vi "Define Schema Name.vi"(11 "Sequence Context":T1) -> (0 "error out":errorcluster, 3 "SchemaName":string)   [LabVIEW 2023, in "HardwareAbstractionLayer_LVOOP.lvlib" / "Report.lvclass"]
uses:
  Report.lvclass
  <vilib>/addons/TestStand/_TSLegacy.llb/LabVIEW Test - Sequence Context.ctl
  Control/Action FGV.ctl
  Control/Result FGV Data.ctl
  <vilib>/Utility/error.llb/Trim Whitespace One-Sided.vi
  <vilib>/addons/TestStand/_TSUtility.llb/TestStand - Get Property Value (String).vi
  <vilib>/addons/TestStand/_TSUtility.llb/TestStand - Set Property Value (String).vi
  <vilib>/addons/TestStand/_TSUtility.llb/TestStand - Set Property Value (Number {Unsigned 32-bit Integer}).vi
  Database/Database.lvclass
  Database/SQL Public VI/Control/DB Options.ctl
panel:
  out "# Total Cycles":u32
  out "# Cycles Completed":u32
  in  "Schema":string(combo)
  in  "Temparature Chamber Name":string
  in  "Test Description":string
  in  "Project Name":string
  out "Date and Time":string
  out "current time":timestamp
  in  "Ok":bool
  in  "Test Phase":string(combo)
  in  "Test Name":string(combo)
  in  "Product Varient":string(combo)
  in  "Product Name":string(combo)
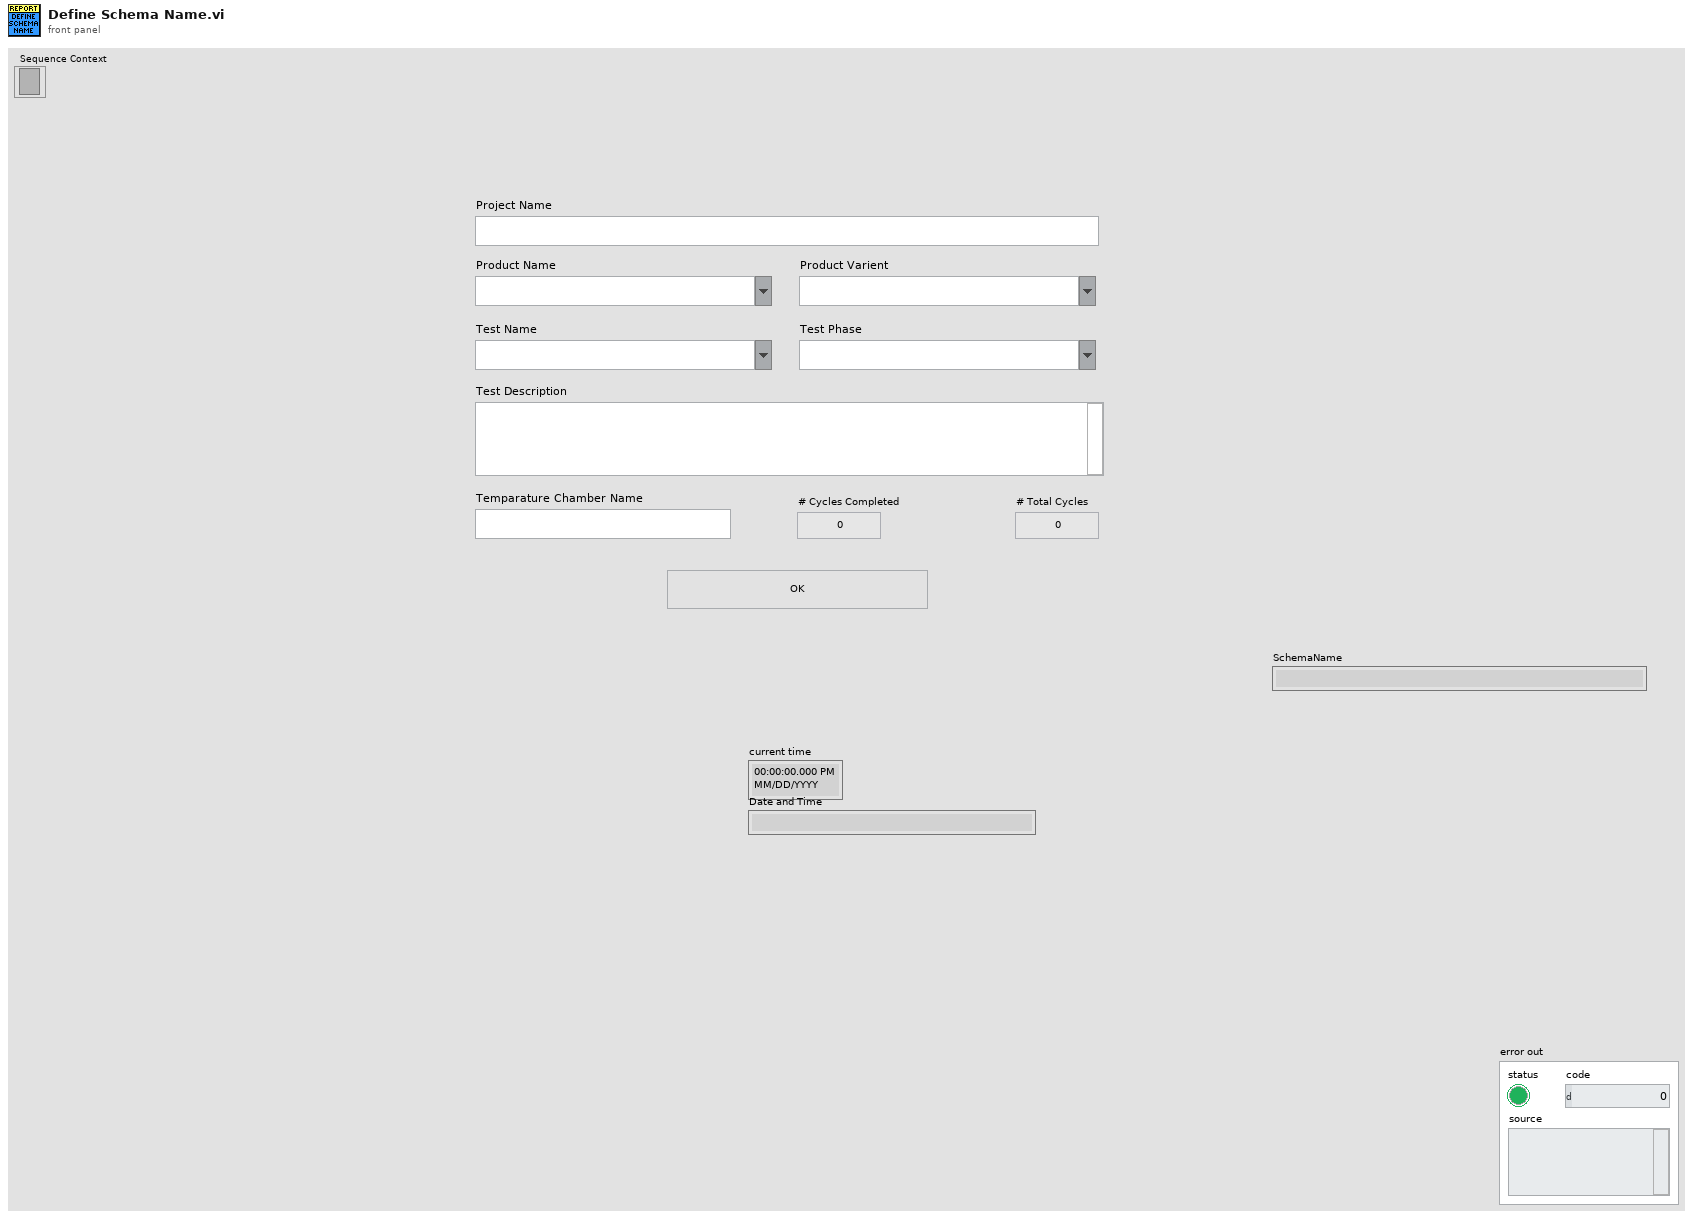
[diagram p1: front panel]
types:
  T1 = typedef "LabVIEW Test - Sequence Context.ctl" = refnum<k7>
  T2 = typedef "HardwareAbstractionLayer_LVOOP.lvlib/Database.lvclass/DB Options.ctl" = enum16{"Init", "Select Data", "Insert Data", "Update Data", "Delete Data", "Execute Query", "Create Schema", "Create Table", "List Tables", "List Columns", "Close"}
  T3 = enum8{"Enabled", "Disabled", "Disabled and Grayed Out"}
  T4 = typedef "HardwareAbstractionLayer_LVOOP.lvlib/Report.lvclass/Result FGV Data.ctl" = cluster{"Project Name":string, "Product Name":string, "Product Varient":string, "Test Name":string, "Test Phase":string, "Test Description":string, "Temp Chamber Name":string, "Schema":string, "Total No of Cycles":u32, "Current Cycle Number":u32, "Cycle Duration":u32, "Current Test Mode":string}
  T5 = typedef "HardwareAbstractionLayer_LVOOP.lvlib/Report.lvclass/Action FGV.ctl" = enum16{"Init", "Set Project Name", "Set Product Name", "Set Product Varient", "Set Test Name", "Set Test Phase", "Set Test Description", "Set Temp Chamber Name", "Set Cycle Duration", "Set Current Cycle Number", "Set Schema", "Set Total No Of Cycle", "Set Current Test Mode", "Set All Data", "Get All Data"}
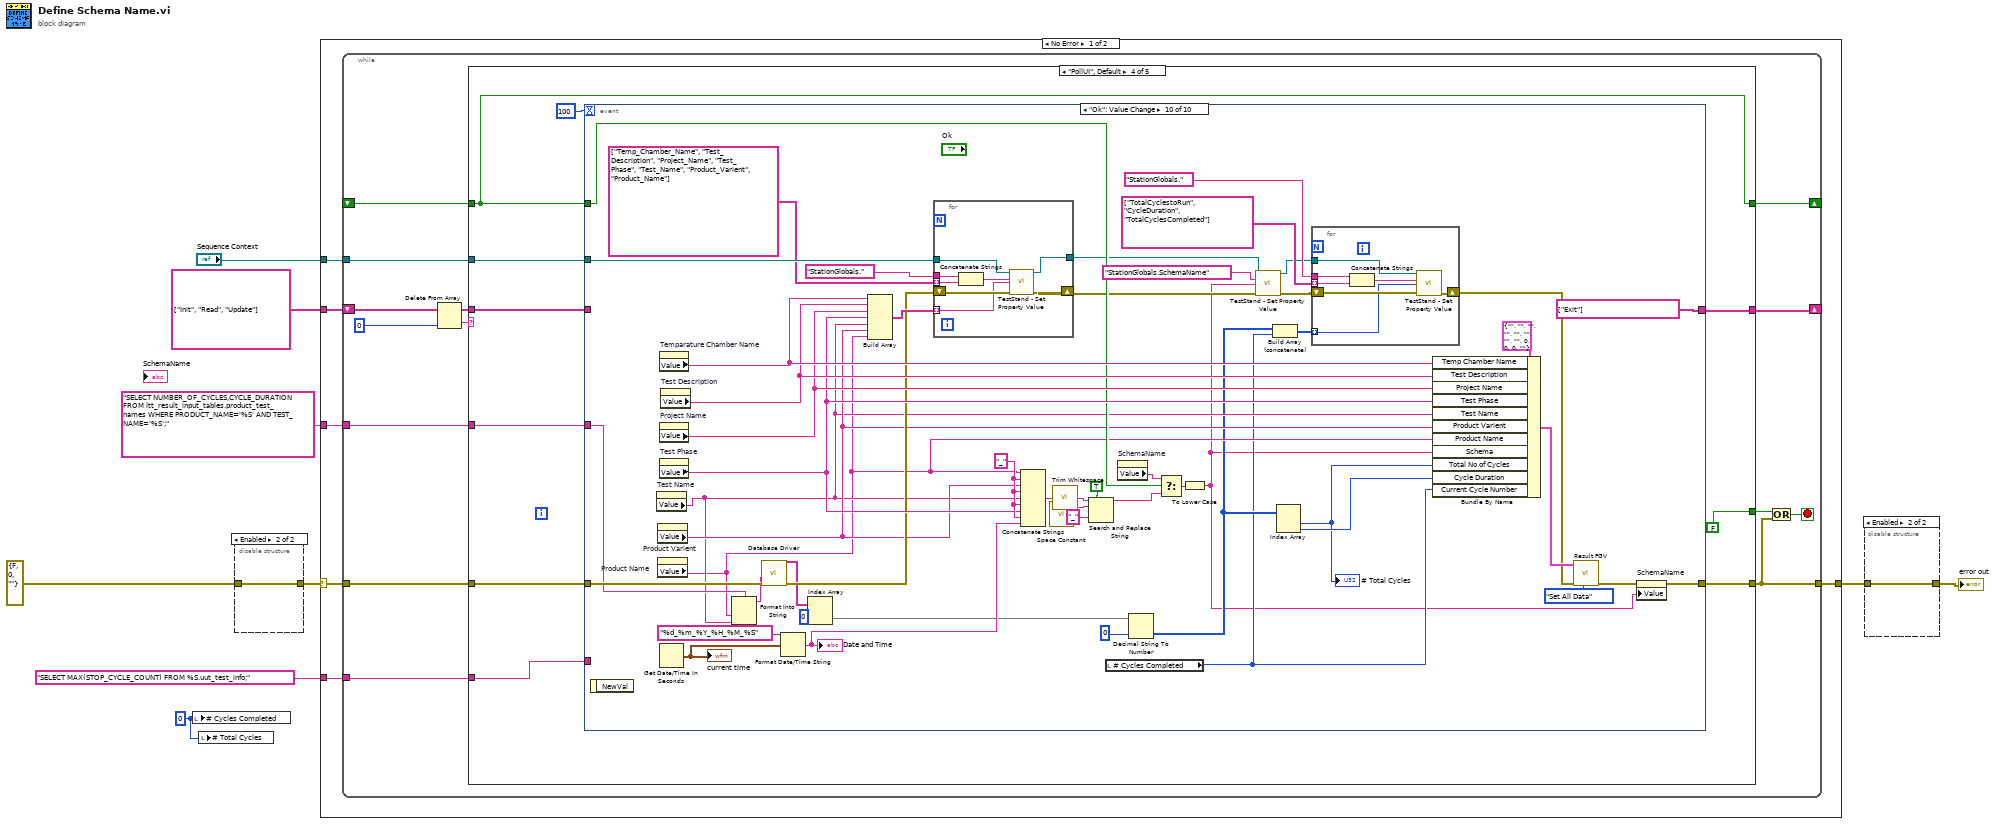
[diagram p0: block diagram]
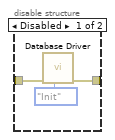
[diagram p2: hidden frame]
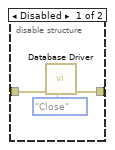
[diagram p3: hidden frame]
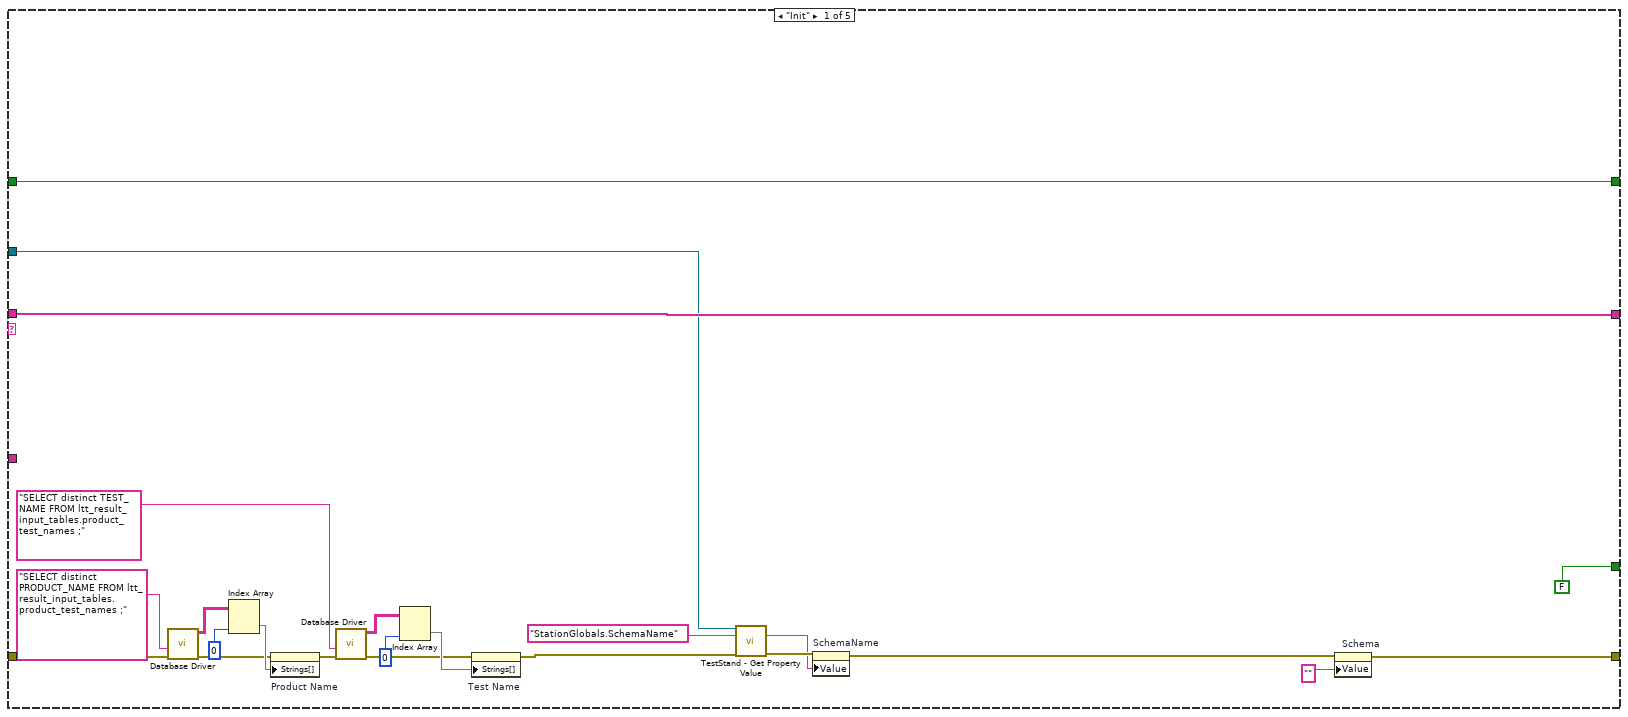
[diagram p4: hidden frame]
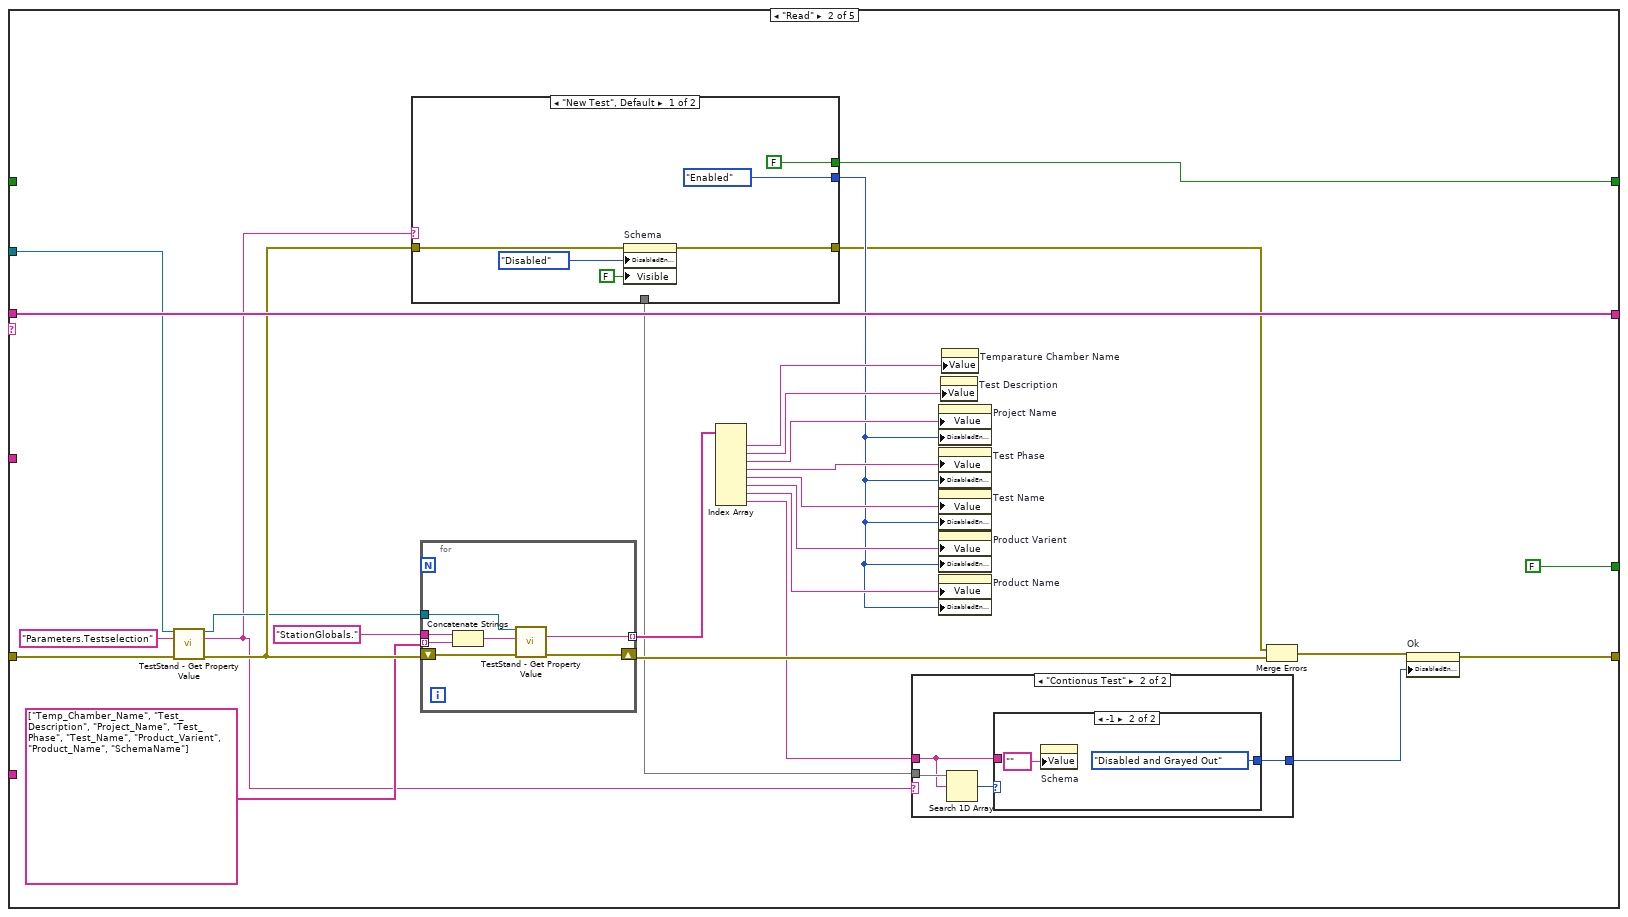
[diagram p5: hidden frame]
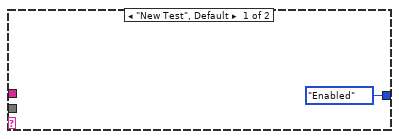
[diagram p6: hidden frame]
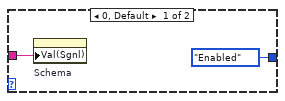
[diagram p7: hidden frame]
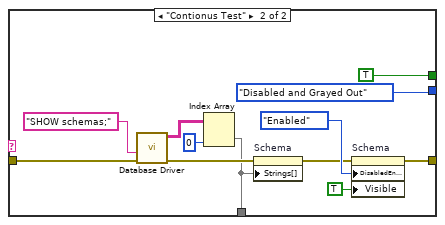
[diagram p8: hidden frame]
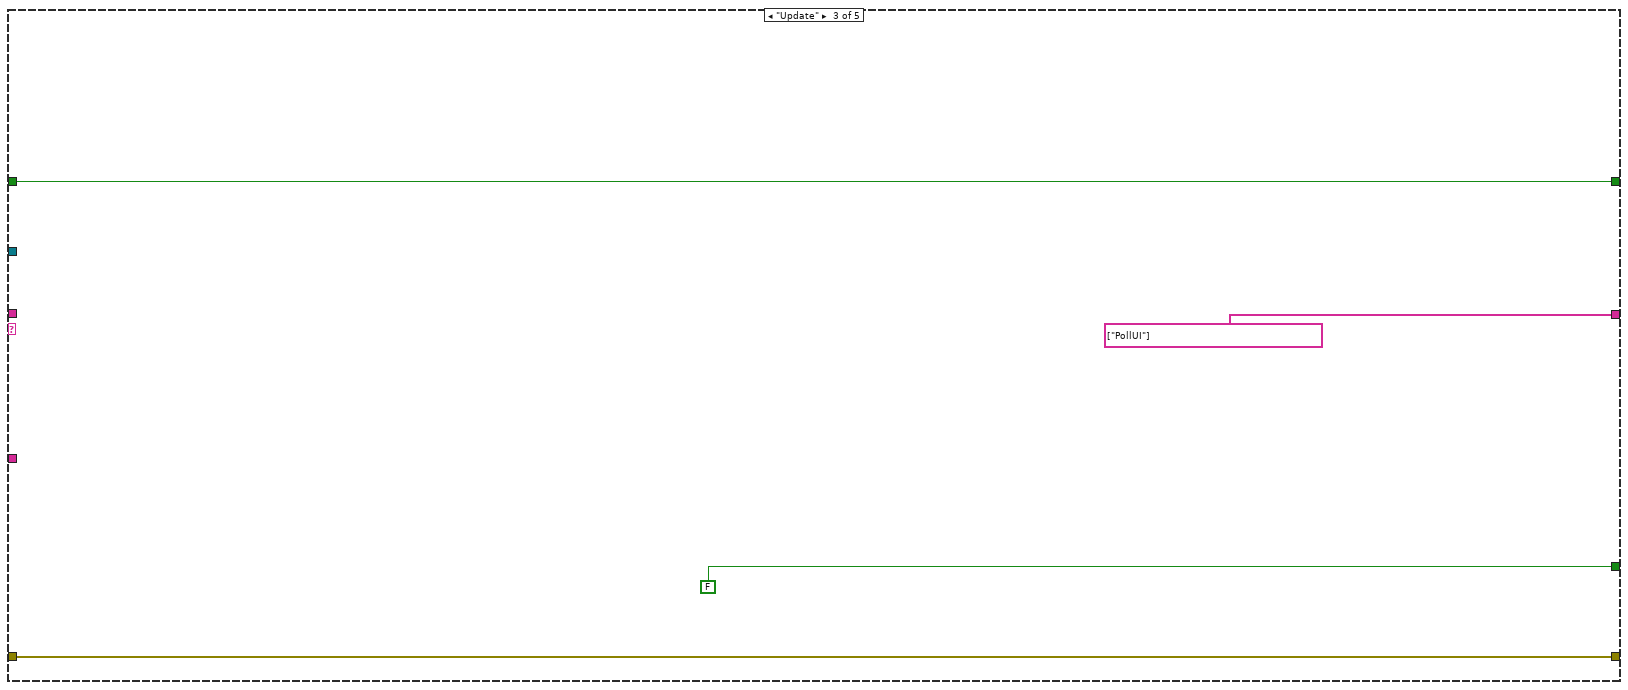
[diagram p9: hidden frame]
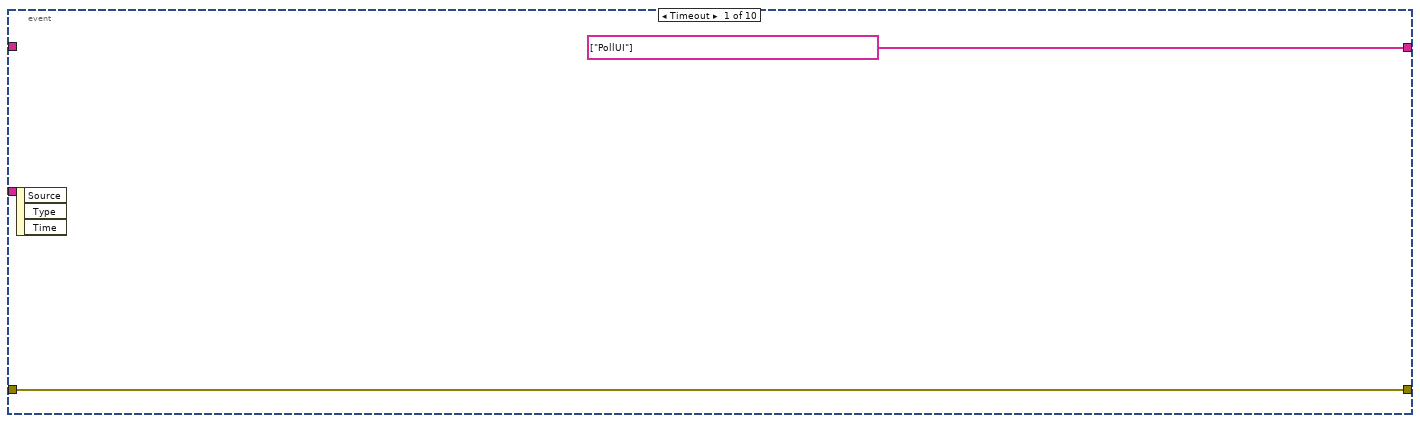
[diagram p10: hidden frame]
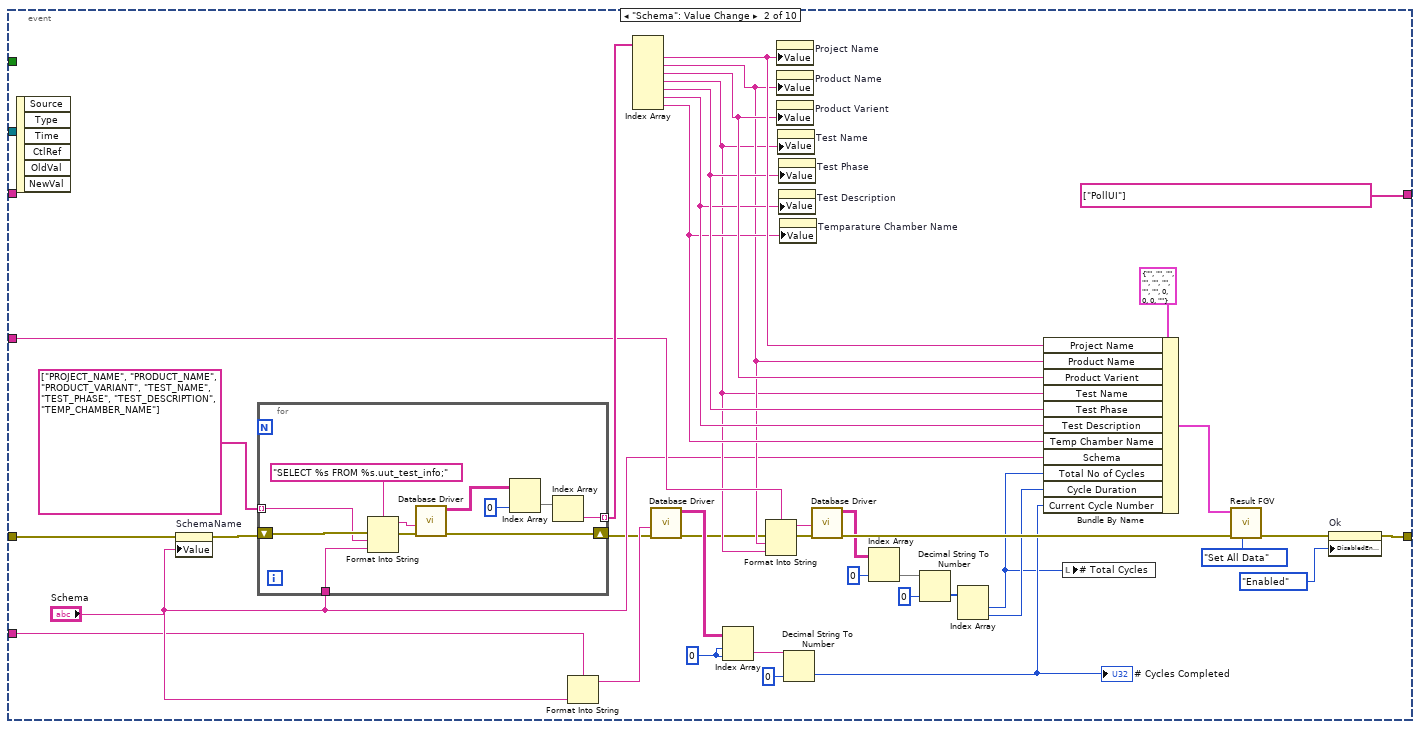
[diagram p11: hidden frame]
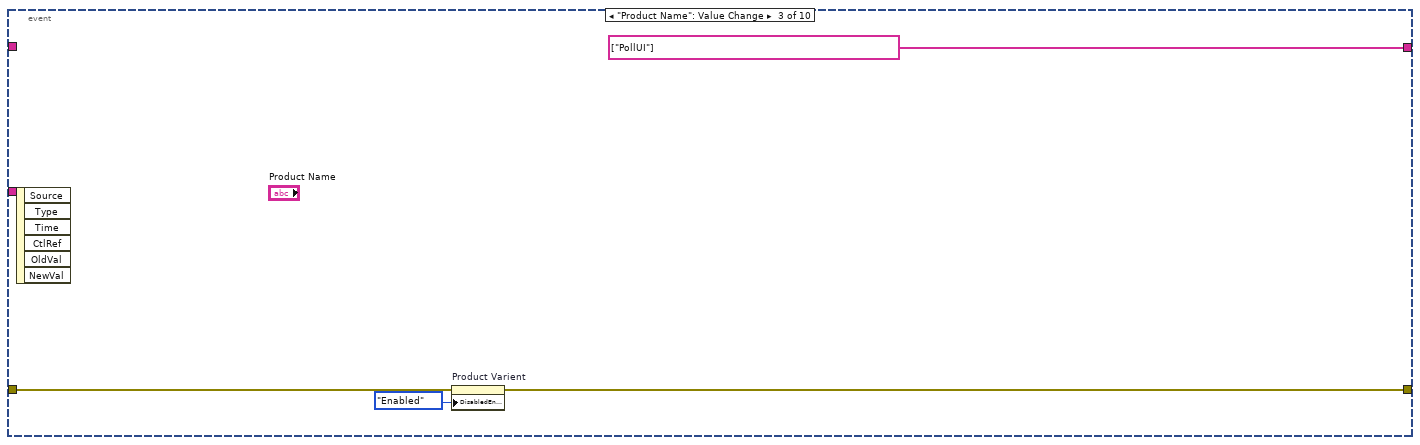
[diagram p12: hidden frame]
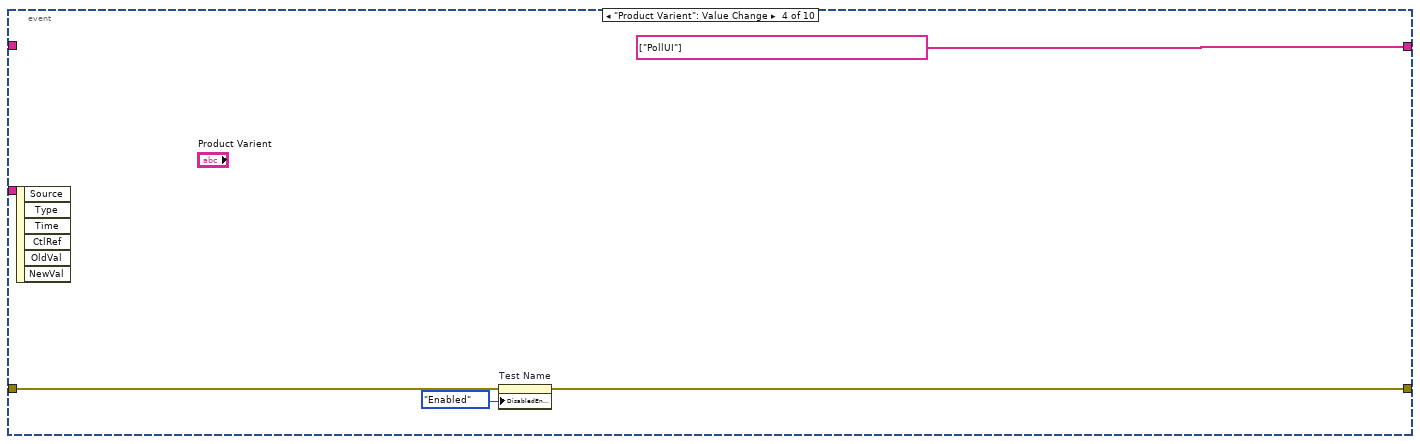
[diagram p13: hidden frame]
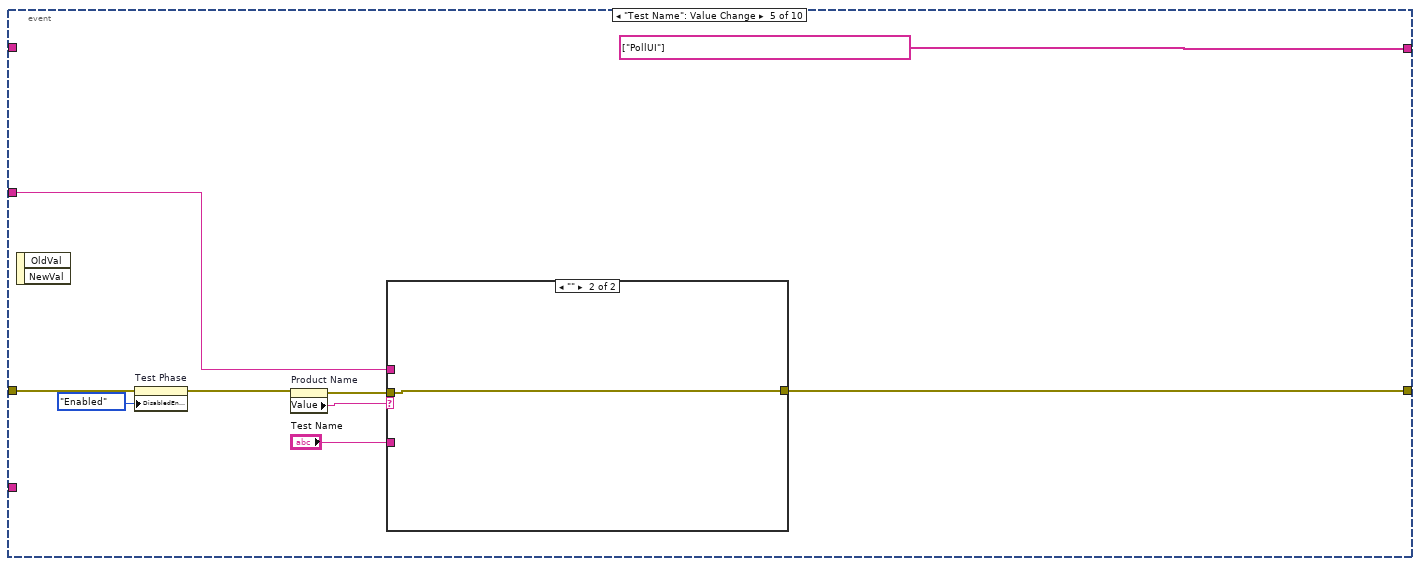
[diagram p14: hidden frame]
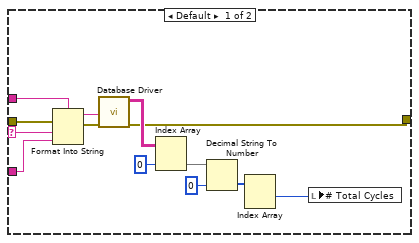
[diagram p15: hidden frame]
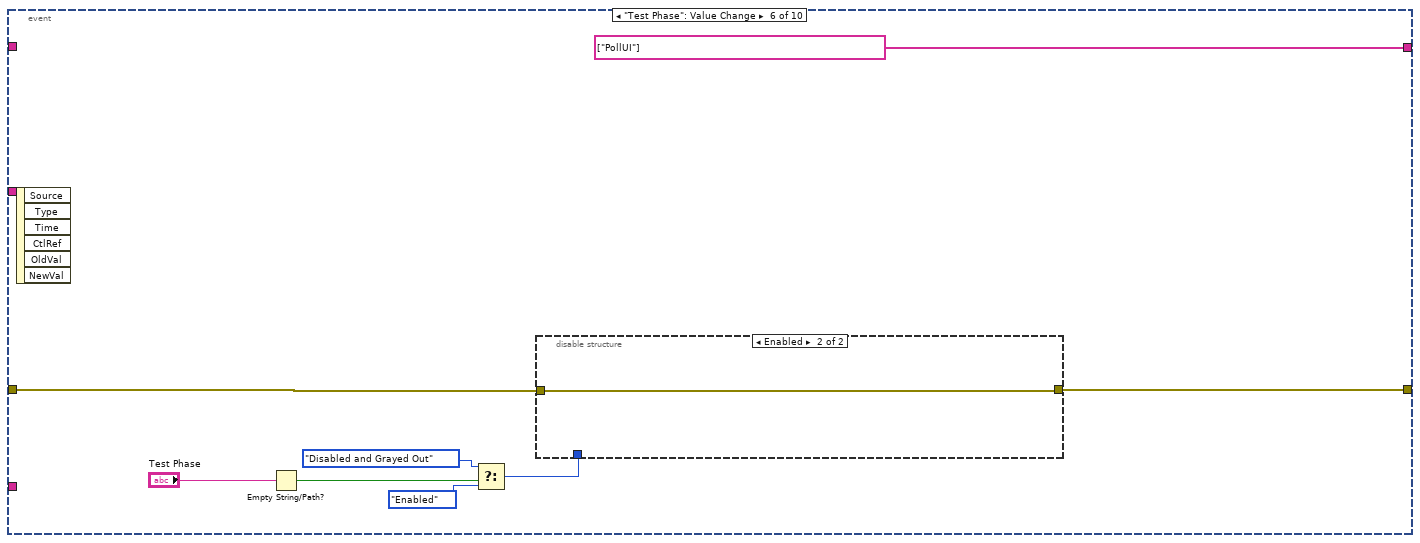
[diagram p16: hidden frame]
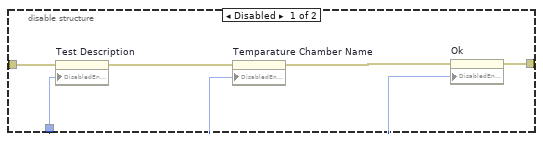
[diagram p17: hidden frame]
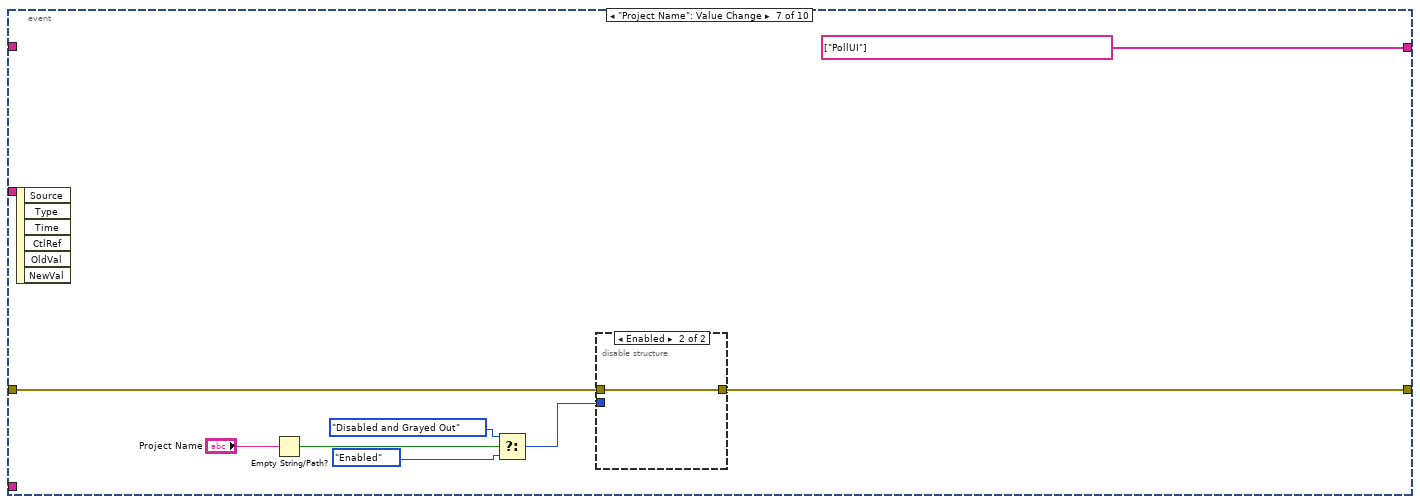
[diagram p18: hidden frame]
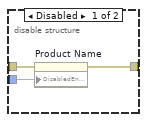
[diagram p19: hidden frame]
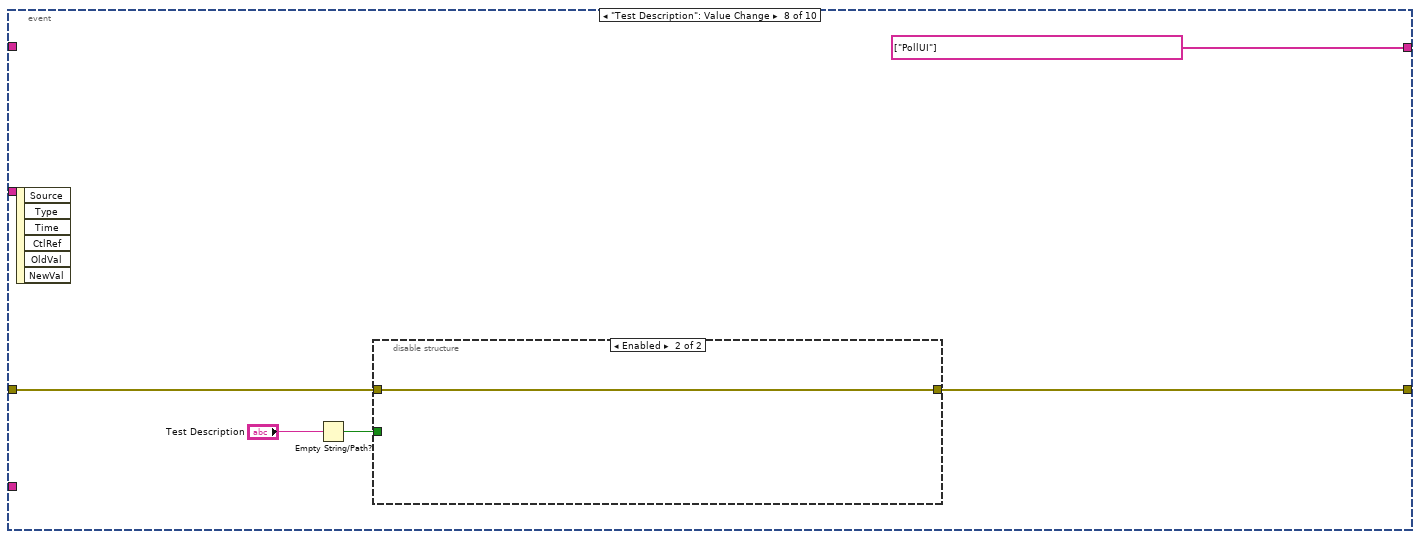
[diagram p20: hidden frame]
diagram:
  w2 = u32 0 ("# Cycles Completed")
  n1 = local write "# Cycles Completed"(w2) -> ()
  n2 = local write "# Total Cycles"(w2) -> ()
  n3 = disable-structure shown="Enabled" {
    disable-tunnel: errorcluster {"status"=FALSE, "code"=0, "source"=""} ("error in") -> [w12 w13]
    disable-tunnel: [w11 w13] -> w9
    frame Disabled {
      n4 = call "Database Driver.vi"("Options"=DB_Options."Init", "error in"=w12) -> ("error out"=w11:errorcluster)  [unwired: 6 in, 3 out]
    }
    frame Enabled {
    }
  }
  n5 = case shown="No Error" w9 {
    selector: w9 -> [w19 w343]
    tunnel: [w18 w343] -> w8
    tunnel: string[] ["Init", "Read", "Update"] -> [w17 _]
    tunnel: "Sequence Context" -> [w16 _]
    tunnel: "SELECT NUMBER_OF_CYCLES,CYCLE_DURATION  FROM ltt_result_input_tables.product_test_names WHERE PRODUCT_NAME='%S' AND TEST_NAME='%S';" -> [w15 _]
    tunnel: "SELECT MAX(STOP_CYCLE_COUNT) FROM %S.uut_test_info;" -> [w14 _]
    frame No Error {
      n6 = while {
        tunnel: w19 -> [w33]
        tunnel: [w26] -> w18
        shift-right: [w29] -> _
        shift-left: w17 -> [w32]
        tunnel: w16 -> [w24]
        shift-right: [w23] -> _
        shift-left: _ -> [w22]
        tunnel: w15 -> [w21]
        tunnel: w14 -> [w20]
        stop <- w27 stop-if-true
        n7 = Delete From Array(array=w32, index=0) -> (deleted portion=w31:string, array with subset deleted=w30:string[])  [unwired: 1 in]
        n8 = case shown="\"PollUI\", Default" w31 {
          tunnel: w33 -> [w53 w80 w119 w130 w333]
          tunnel: [w37 w60 w119 w129 w332] -> w26
          tunnel: w30 -> [w56 w83 _ w128 _]
          tunnel: [w56 w83 string[] ["PollUI"] w127 string[] ["Exit"]] -> w29
          tunnel: [FALSE FALSE FALSE FALSE TRUE] -> w28
          tunnel: w24 -> [w36 w81 _ w125 w338]
          tunnel: [w42 w70 w118 w124 w340] -> w23
          tunnel: w22 -> [w42 _ w118 w124 w340]
          tunnel: w21 -> [_ _ _ w123 _]
          tunnel: w20 -> [_ _ _ w122 _]
          frame "Init" {
            n9 = call "Database Driver.vi"("error in"=w53, "SQL query"="SELECT distinct PRODUCT_NAME FROM ltt_result_input_tables.product_test_names ;") -> ("error out"=w49:errorcluster, "data"=w52:string[][])  [unwired: 6 in, 2 out]
            n10 = Index Array(array=w52, index (col)=0 ("disabled index (col)")) -> (element=w50:string[])  [unwired: 1 in]
            n11 = property on="Product Name" class="CmbBox"(error in=w49, "Strings[]"=w50) -> (error out=w45:errorcluster)  [unwired: 1 in, 1 out]
            n12 = call "Database Driver.vi"("error in"=w45, "SQL query"="SELECT distinct TEST_NAME FROM ltt_result_input_tables.product_test_names ;") -> ("error out"=w44:errorcluster, "data"=w47:string[][])  [unwired: 6 in, 2 out]
            n13 = Index Array(array=w47, index (col)=0 ("disabled index (col)")) -> (element=w46:string[])  [unwired: 1 in]
            n14 = property on="Test Name" class="CmbBox"(error in=w44, "Strings[]"=w46) -> (error out=w41:errorcluster)  [unwired: 1 in, 1 out]
            n15 = call-poly <vilib>:"TestStand - Get Property Value.vi"("Sequence Context In"=w36, "Lookup String"="StationGlobals.SchemaName", "error in (no error)"=w41) -> ("Value"=w38:string, "error out"=w39:errorcluster)  [unwired: 10 in, 1 out]
            n16 = property on="SchemaName" class="Str"(error in=w39, "Value"=w38) -> (error out=w35:errorcluster)  [unwired: 1 in, 1 out]
            n17 = property on="Schema" class="CmbBox"(error in=w35, "Value"="" ("Value (Signaling)")) -> (error out=w37:errorcluster)  [unwired: 1 in, 1 out]
          }
          frame "Read" {
            n18 = call-poly <vilib>:"TestStand - Get Property Value.vi"("Sequence Context In"=w81, "Lookup String"="Parameters.Testselection", "error in (no error)"=w80) -> ("Sequence Context Out"=w63:refnum<k7>, "Value"=w59:string, "error out"=w69:errorcluster)  [unwired: 10 in]
            n19 = case shown="\"New Test\", Default" w59 {
              tunnel: [T3."Enabled" ("Disabled") T3."Disabled and Grayed Out" ("Disabled")] -> w71
              tunnel: [FALSE TRUE] -> w70
              tunnel: w69 -> [w102 w112]
              tunnel: [w101 w108] -> w67
              tunnel: [_ w106] -> w58
              frame "New Test", Default {
                n20 = property on="Schema" class="CmbBox"(error in=w102, "DisabledEnum"=T3."Disabled" ("Disabled"), "Visible"=FALSE) -> (error out=w101:errorcluster)  [unwired: 1 in, 1 out]
              }
              frame "Contionus Test" {
                n21 = call "Database Driver.vi"("error in"=w112, "SQL query"="SHOW schemas;") -> ("error out"=w111:errorcluster, "data"=w115:string[][])  [unwired: 6 in, 2 out]
                n22 = Index Array(array=w115, index (col)=0 ("disabled index (col)")) -> (element=w106:string[])  [unwired: 1 in]
                n23 = property on="Schema" class="CmbBox"(error in=w111, "Strings[]"=w106) -> (error out=w109:errorcluster)  [unwired: 1 in, 1 out]
                n24 = property on="Schema" class="CmbBox"(error in=w109, "DisabledEnum"=T3."Enabled" ("Disabled"), "Visible"=TRUE) -> (error out=w108:errorcluster)  [unwired: 1 in, 1 out]
              }
            }
            n25 = for {
              tunnel: "StationGlobals." -> [w99]
              tunnel: string[] ["Temp_Chamber_Name", "Test_Description", "Project_Name", "Test_Phase", "Test_Name", "Product_Varient", "Product_Name", "SchemaName"] -> [w98] mode=indexing
              tunnel: w63 -> [w95]
              tunnel: [w94] -> w79 mode=indexing
              shift-right: [w93] -> w62
              shift-left: w69 -> [w96]
              n26 = Concatenate Strings(w99, w98) -> (w97:string)
              n27 = call-poly <vilib>:"TestStand - Get Property Value.vi"("Sequence Context In"=w95, "Lookup String"=w97, "error in (no error)"=w96) -> ("Value"=w94:string, "error out"=w93:errorcluster)  [unwired: 10 in, 1 out]
            }
            n28 = Index Array(array=w79) -> (element #1=w78:string, element #2=w77:string, element #3=w76:string, element #4=w75:string, element #5=w74:string, element #6=w73:string, element #7=w72:string, element #8=w61:string)  [unwired: 8 in]
            n29 = case shown="\"Contionus Test\"" w59 {
              tunnel: w61 -> [_ w87]
              tunnel: w58 -> [_ w88]
              tunnel: [T3."Enabled" ("Disabled") w85] -> w57
              frame "New Test", Default {
              }
              frame "Contionus Test" {
                n30 = Search 1D Array(1D array=w88, element=w87) -> (index of element=w86:i32)  [unwired: 1 in]
                n31 = case shown="-1" w86 {
                  tunnel: w87 -> [w90 _]
                  tunnel: [T3."Enabled" ("Disabled") T3."Disabled and Grayed Out" ("Disabled")] -> w85
                  frame 0, Default {
                    n32 = property on="Schema" class="CmbBox"("Val(Sgnl)"=w90) -> ()  [unwired: 2 in, 2 out]
                  }
                  frame -1 {
                    n33 = property on="Schema" class="CmbBox"("Value"="" ("Schema")) -> ()  [unwired: 2 in, 2 out]
                  }
                }
              }
            }
            n34 = property on="Project Name" class="Str"("Value"=w76, "DisabledEnum"=w71) -> ()  [unwired: 2 in, 2 out]
            n35 = property on="Test Phase" class="CmbBox"("Value"=w75, "DisabledEnum"=w71) -> ()  [unwired: 2 in, 2 out]
            n36 = property on="Test Name" class="CmbBox"("Value"=w74, "DisabledEnum"=w71) -> ()  [unwired: 2 in, 2 out]
            n37 = property on="Product Varient" class="CmbBox"("Value"=w73, "DisabledEnum"=w71) -> ()  [unwired: 2 in, 2 out]
            n38 = property on="Product Name" class="CmbBox"("Value"=w72, "DisabledEnum"=w71) -> ()  [unwired: 2 in, 2 out]
            n39 = property on="Test Description" class="Str"("Value"=w77) -> ()  [unwired: 2 in, 2 out]
            n40 = property on="Temparature Chamber Name" class="Str"("Value"=w78) -> ()  [unwired: 2 in, 2 out]
            n41 = Merge Errors(w67, w62) -> (w68:errorcluster)
            n42 = property on="Ok" class="Bool"(error in=w68, "DisabledEnum"=w57) -> (error out=w60:errorcluster)  [unwired: 1 in, 1 out]
          }
          frame "Update" {
          }
          frame "PollUI", Default {
            n43 = event shown="[9] \"Ok\": Value Change" {
              selector: _ -> [_ _ _ _ _ _ _ _ _ _]
              dyn-events: _ -> [_ _ _ _ _ _ _ _ _ _]
              timeout: 100 -> [_ _ _ _ _ _ _ _ _ _]
              tunnel: w130 -> [w133 w171 w185 w189 w198 w221 w234 w242 w254 w288]
              tunnel: [w133 w135 w184 w188 w192 w216 w233 w241 w253 w289] -> w129
              tunnel: [string[] ["PollUI"] string[] ["PollUI"] string[] ["PollUI"] string[] ["PollUI"] string[] ["PollUI"] string[] ["PollUI"] string[] ["PollUI"] string[] ["PollUI"] string[] ["PollUI"] string[] ["Exit"]] -> w127
              tunnel: w128 -> [_ _ _ _ _ _ _ _ _ _]
              tunnel: w125 -> [_ _ _ _ _ _ _ _ _ w303]
              tunnel: w124 -> [_ _ _ _ _ _ _ _ _ w296]
              tunnel: w123 -> [_ w157 _ _ w196 _ _ _ _ w285]
              tunnel: w122 -> [_ w139 _ _ _ _ _ _ _ _]
              event Timeout {
                n44 = event-data() -> ()  [unwired: 1 in, 3 out]
              }
              event "Schema": Value Change {
                w140 = 0 ("disabled index (col)")
                n45 = event-data() -> ()  [unwired: 1 in, 6 out]
                n46 = property on="SchemaName" class="Str"(error in=w171, "Value"="Schema") -> (error out=w168:errorcluster)  [unwired: 1 in, 1 out]
                n47 = for {
                  tunnel: "Schema" -> [w178]
                  shift-right: [w175] -> w142
                  shift-left: w168 -> [w177]
                  tunnel: string[] ["PROJECT_NAME", "PRODUCT_NAME", "PRODUCT_VARIANT", "TEST_NAME", "TEST_PHASE", "TEST_DESCRIPTION", "TEMP_CHAMBER_NAME"] -> [w174] mode=indexing
                  tunnel: [w173] -> w166 mode=indexing
                  n48 = Format Into String(format string="SELECT %s FROM %s.uut_test_info;", error in=w177, w174, w178) -> (resulting string=w179:string, error out=w176:errorcluster)  [unwired: 1 in]
                  n49 = call "Database Driver.vi"("error in"=w176, "SQL query"=w179) -> ("error out"=w175:errorcluster, "data"=w183:string[][])  [unwired: 6 in, 2 out]
                  n50 = Index Array(array=w183, index (col)=0 ("disabled index (col)")) -> (element=w181:string[])  [unwired: 1 in]
                  n51 = Index Array(array=w181) -> (element=w173:string)  [unwired: 1 in]
                }
                n52 = Format Into String(format string=w139, "Schema") -> (resulting string=w146:string)  [unwired: 2 in, 1 out]
                n53 = Index Array(array=w166) -> (element #1=w164:string, element #2=w149:string, element #3=w163:string, element #4=w148:string, element #5=w162:string, element #6=w161:string, element #7=w160:string)  [unwired: 7 in]
                n54 = call "Database Driver.vi"("error in"=w142, "SQL query"=w146) -> ("error out"=w141:errorcluster, "data"=w145:string[][])  [unwired: 6 in, 2 out]
                n55 = Index Array(array=w145, index (row)=w140, index (col)=w140) -> (element=w144:string)
                n56 = Format Into String(format string=w157, error in=w141, w149, w148) -> (resulting string=w155:string, error out=w156:errorcluster)  [unwired: 1 in]
                n57 = property on="Project Name" class="Str"("Value"=w164) -> ()  [unwired: 2 in, 2 out]
                n58 = property on="Product Name" class="CmbBox"("Value"=w149) -> ()  [unwired: 2 in, 2 out]
                n59 = property on="Product Varient" class="CmbBox"("Value"=w163) -> ()  [unwired: 2 in, 2 out]
                n60 = property on="Test Name" class="CmbBox"("Value"=w148) -> ()  [unwired: 2 in, 2 out]
                n61 = property on="Test Phase" class="CmbBox"("Value"=w162) -> ()  [unwired: 2 in, 2 out]
                n62 = property on="Test Description" class="Str"("Value"=w161) -> ()  [unwired: 2 in, 2 out]
                n63 = property on="Temparature Chamber Name" class="Str"("Value"=w160) -> ()  [unwired: 2 in, 2 out]
                n64 = Decimal String To Number(string=w144, default (0L)=u32 0 ("default (0 I32)")) -> (number=w138:u32)  [unwired: 1 in, 1 out]
                "# Cycles Completed" <- w138
                n65 = call "Database Driver.vi"("error in"=w156, "SQL query"=w155) -> ("error out"=w154:errorcluster, "data"=w153:string[][])  [unwired: 6 in, 2 out]
                n66 = Index Array(array=w153, index (col)=0 ("disabled index (col)")) -> (element=w152:string[])  [unwired: 1 in]
                n67 = Decimal String To Number(string=w152, default (0L)=u32 0 ("default (0 I32)")) -> (number=w151:u32[])  [unwired: 1 in, 1 out]
                n68 = Index Array(array=w151) -> (element #1=w137:u32, element #2=w150:u32)  [unwired: 2 in]
                n69 = Bundle By Name(cluster=T4 {"Project Name"="", "Product Name"="", "Product Varient"="", "Test Name"="", "Test Phase"="", "Test Description"="", "Temp Chamber Name"="", "Schema"="", "Total No of Cycles"=0, "Current Cycle Number"=0, "Cycle Duration"=0, "Current Test Mode"=""} ("Result FGV Data In"), "Project Name"=w164, "Product Name"=w149, "Product Varient"=w163, "Test Name"=w148, "Test Phase"=w162, "Test Description"=w161, "Temp Chamber Name"=w160, "Schema"="Schema", "Total No of Cycles"=w137, "Cycle Duration"=w150, "Current Cycle Number"=w138) -> (w170:T4)
                n70 = local write "# Total Cycles"(w137) -> ()
                n71 = call "Result FGV.vi"("Action(Get All Data)"=Action_FGV."Set All Data", "error in"=w154, "Result FGV Data In"=w170) -> ("error out"=w136:errorcluster)  [unwired: 7 in, 1 out]
                n72 = property on="Ok" class="Bool"(error in=w136, "DisabledEnum"=T3."Enabled" ("Disabled")) -> (error out=w135:errorcluster)  [unwired: 1 in, 1 out]
              }
              event "Product Name": Value Change {
                n73 = event-data() -> ()  [unwired: 1 in, 6 out]
                n74 = property on="Product Varient" class="CmbBox"(error in=w185, "DisabledEnum"=T3."Enabled" ("Disabled")) -> (error out=w184:errorcluster)  [unwired: 1 in, 1 out]
              }
              event "Product Varient": Value Change {
                n75 = event-data() -> ()  [unwired: 1 in, 6 out]
                n76 = property on="Test Name" class="CmbBox"(error in=w189, "DisabledEnum"=T3."Enabled" ("Disabled")) -> (error out=w188:errorcluster)  [unwired: 1 in, 1 out]
              }
              event "Test Name": Value Change {
                n77 = event-data() -> ()  [unwired: 1 in, 2 out]
                n78 = property on="Test Phase" class="CmbBox"(error in=w198, "DisabledEnum"=T3."Enabled" ("Disabled")) -> (error out=w195:errorcluster)  [unwired: 1 in, 1 out]
                n79 = property on="Product Name" class="CmbBox"(error in=w195) -> (error out=w194:errorcluster, "Value"=w197:string)  [unwired: 1 in, 1 out]
                n80 = case shown="\"\"" w197 {
                  selector: w197 -> [w206 _]
                  tunnel: w196 -> [w205 _]
                  tunnel: w194 -> [w204 w214]
                  tunnel: "Test Name" -> [w203 _]
                  tunnel: [w202 w214] -> w192
                  frame Default {
                    n81 = Format Into String(format string=w205, error in=w204, w206, w203) -> (resulting string=w210:string, error out=w211:errorcluster)  [unwired: 1 in]
                    n82 = call "Database Driver.vi"("error in"=w211, "SQL query"=w210) -> ("error out"=w202:errorcluster, "data"=w209:string[][])  [unwired: 6 in, 2 out]
                    n83 = Index Array(array=w209, index (col)=0 ("disabled index (col)")) -> (element=w208:string[])  [unwired: 1 in]
                    n84 = Decimal String To Number(string=w208, default (0L)=u32 0 ("default (0 I32)")) -> (number=w207:u32[])  [unwired: 1 in, 1 out]
                    n85 = Index Array(array=w207) -> (element #1=w201:u32)  [unwired: 2 in, 1 out]
                    n86 = local write "# Total Cycles"(w201) -> ()
                  }
                  frame "" {
                  }
                }
              }
              event "Test Phase": Value Change {
                n87 = event-data() -> ()  [unwired: 1 in, 6 out]
                n88 = Empty String/Path?(string/path="Test Phase") -> (empty?=w219:bool)
                n89 = Select(t=T3."Disabled and Grayed Out" ("Disabled"), s=w219, f=T3."Enabled") -> (s? t:f=w215:T3)
                n90 = disable-structure shown="Enabled" {
                  disable-tunnel: w221 -> [w227 w228]
                  disable-tunnel: [w224 w228] -> w216
                  disable-tunnel: w215 -> [w223 _]
                  frame Disabled {
                    n91 = property on="Test Description" class="Str"(error in=w227, "DisabledEnum"=w223) -> (error out=w226:errorcluster)  [unwired: 1 in, 1 out]
                    n92 = property on="Temparature Chamber Name" class="Str"(error in=w226, "DisabledEnum"=w223) -> (error out=w225:errorcluster)  [unwired: 1 in, 1 out]
                    n93 = property on="Ok" class="Bool"(error in=w225, "DisabledEnum"=w223) -> (error out=w224:errorcluster)  [unwired: 1 in, 1 out]
                  }
                  frame Enabled {
                  }
                }
              }
              event "Project Name": Value Change {
                n94 = event-data() -> ()  [unwired: 1 in, 6 out]
                n95 = Empty String/Path?(string/path="Project Name") -> (empty?=w231:bool)
                n96 = Select(t=T3."Disabled and Grayed Out" ("Disabled"), s=w231, f=T3."Enabled" ("Disabled")) -> (s? t:f=w230:T3)
                n97 = disable-structure shown="Enabled" {
                  disable-tunnel: w234 -> [w239 w240]
                  disable-tunnel: [w238 w240] -> w233
                  disable-tunnel: w230 -> [w237 _]
                  frame Disabled {
                    n98 = property on="Product Name" class="CmbBox"(error in=w239, "DisabledEnum"=w237) -> (error out=w238:errorcluster)  [unwired: 1 in, 1 out]
                  }
                  frame Enabled {
                  }
                }
              }
              event "Test Description": Value Change {
                n99 = event-data() -> ()  [unwired: 1 in, 6 out]
                n100 = Empty String/Path?(string/path="Test Description") -> (empty?=w243:bool)
                n101 = disable-structure shown="Enabled" {
                  disable-tunnel: w243 -> [w251 _]
                  disable-tunnel: w242 -> [w248 w252]
                  disable-tunnel: [w247 w252] -> w241
                  frame Disabled {
                    n102 = Select(t=T3."Disabled and Grayed Out" ("Disabled"), s=w251, f=T3."Enabled" ("Disabled")) -> (s? t:f=w246:T3)
                    n103 = property on="Temparature Chamber Name" class="Str"(error in=w248, "DisabledEnum"=w246) -> (error out=w247:errorcluster)  [unwired: 1 in, 1 out]
                  }
                  frame Enabled {
                  }
                }
              }
              event "Temparature Chamber Name": Value Change {
                n104 = event-data() -> ()  [unwired: 1 in, 6 out]
                n105 = Empty String/Path?(string/path="Temparature Chamber Name") -> (empty?=w255:bool)
                n106 = disable-structure shown="Enabled" {
                  disable-tunnel: w255 -> [w263 _]
                  disable-tunnel: w254 -> [w259 w264]
                  disable-tunnel: [w258 w264] -> w253
                  frame Disabled {
                    n107 = Select(t=T3."Disabled and Grayed Out" ("Disabled"), s=w263, f=T3."Enabled" ("Disabled")) -> (s? t:f=w261:T3)
                    n108 = property on="Ok" class="Bool"(error in=w259, "DisabledEnum"=w261) -> (error out=w258:errorcluster)  [unwired: 1 in, 1 out]
                  }
                  frame Enabled {
                  }
                }
              }
              event "Ok": Value Change {
                w312 = "_"
                n109 = event-data() -> ()  [unwired: 1 in, 1 out]
                n110 = property on="Test Name" class="CmbBox"() -> ("Value"=w283:string)  [unwired: 2 in, 2 out]
                n111 = property on="Product Varient" class="CmbBox"() -> ("Value"=w284:string)  [unwired: 2 in, 2 out]
                n112 = property on="Product Name" class="CmbBox"() -> ("Value"=w280:string)  [unwired: 2 in, 2 out]
                n113 = property on="Temparature Chamber Name" class="Str"() -> ("Value"=w301:string)  [unwired: 2 in, 2 out]
                n114 = property on="Project Name" class="Str"() -> ("Value"=w299:string)  [unwired: 2 in, 2 out]
                n115 = property on="Test Phase" class="CmbBox"() -> ("Value"=w297:string)  [unwired: 2 in, 2 out]
                n116 = Get Date/Time In Seconds() -> (seconds since 1Jan1904=w315:timestamp)
                "current time" <- w315
                n117 = property on="Test Description" class="Str"() -> ("Value"=w300:string)  [unwired: 2 in, 2 out]
                n118 = Format Into String(format string=w285, w280, w283) -> (resulting string=w286:string)  [unwired: 2 in, 1 out]
                n119 = call "Database Driver.vi"("error in"=w288, "SQL query"=w286) -> ("error out"=w287:errorcluster, "data"=w282:string[][])  [unwired: 6 in, 2 out]
                n120 = Format Date/Time String(time format string (%c)="%d_%m_%Y_%H_%M_%S", seconds (now)=w315) -> (date/time string=w313:string)  [unwired: 1 in]
                "Date and Time" <- w313
                n121 = Index Array(array=w282, index (row)=0 ("disabled index (col)")) -> (element=w279:string[])  [unwired: 1 in]
                n122 = Build Array(w301, w300, w299, w297, w283, w284, w280) -> (w298:string[])
                n123 = for {
                  tunnel: "StationGlobals." -> [w331]
                  tunnel: string[] ["Temp_Chamber_Name", "Test_Description", "Project_Name", "Test_Phase", "Test_Name", "Product_Varient", "Product_Name"] -> [w330] mode=indexing
                  tunnel: w303 -> [w327]
                  shift-right: [w326] -> w292
                  shift-left: w287 -> [w328]
                  tunnel: w298 -> [w325] mode=indexing
                  tunnel: [w324] -> w293
                  n124 = Concatenate Strings(w331, w330) -> (w329:string)
                  n125 = call-poly <vilib>:"TestStand - Set Property Value.vi"("Sequence Context In"=w327, "Lookup String"=w329, "New Value"=w325, "error in (no error)"=w328) -> ("Sequence Context Out"=w324:refnum<k7>, "error out"=w326:errorcluster)  [unwired: 10 in]
                }
                n126 = Concatenate Strings(w280, w312, w284, w312, w283, w312, w297, w312, w313) -> (w310:string)
                n127 = call <vilib>:"Space Constant.vi"() -> ("String"=w308:string)
                n128 = call <vilib>:"Trim Whitespace.vi"("string"=w310) -> ("trimmed string"=w306:string)  [unwired: 1 in]
                n129 = Search and Replace String(replace all?=TRUE ("replace all? (F)"), input string=w306, search string=w308, replace string="_" ("replace string (\"\")")) -> (result string=w295:string)  [unwired: 4 in, 3 out]
                n130 = local read "# Cycles Completed"() -> (w268:u32)
                n131 = property on="SchemaName" class="Str"() -> ("Value"=w291:string)  [unwired: 2 in, 2 out]
                n132 = Decimal String To Number(string=w279, default (0L)=u32 0 ("default (0 I32)")) -> (number=w270:u32[])  [unwired: 1 in, 1 out]
                n133 = Select(t=w291, s=w296, f=w295) -> (s? t:f=w266:string)
                n134 = To Lower Case(string=w266) -> (all lower case string=w265:string)
                n135 = call-poly <vilib>:"TestStand - Set Property Value.vi"("Sequence Context In"=w293, "Lookup String"="StationGlobals.SchemaName", "New Value"=w265, "error in (no error)"=w292) -> ("Sequence Context Out"=w272:refnum<k7>, "error out"=w273:errorcluster)  [unwired: 10 in]
                n136 = Build Array (concatenate)(w270, w268) -> (w269:u32[])
                n137 = Index Array(array=w270) -> (element #1=w267:u32, element #2=w278:u32)  [unwired: 2 in]
                "# Total Cycles" <- w267
                n138 = for {
                  tunnel: "StationGlobals." -> [w323]
                  tunnel: string[] ["TotalCyclestoRun", "CycleDuration", "TotalCyclesCompleted"] -> [w322] mode=indexing
                  tunnel: w272 -> [w319]
                  shift-right: [w318] -> w271
                  shift-left: w273 -> [w320]
                  tunnel: w269 -> [w317] mode=indexing
                  n139 = Concatenate Strings(w323, w322) -> (w321:string)
                  n140 = call-poly <vilib>:"TestStand - Set Property Value.vi"("Sequence Context In"=w319, "Lookup String"=w321, "New Value"=w317, "error in (no error)"=w320) -> ("error out"=w318:errorcluster)  [unwired: 10 in, 1 out]
                }
                n141 = Bundle By Name(cluster=T4 {"Project Name"="", "Product Name"="", "Product Varient"="", "Test Name"="", "Test Phase"="", "Test Description"="", "Temp Chamber Name"="", "Schema"="", "Total No of Cycles"=0, "Current Cycle Number"=0, "Cycle Duration"=0, "Current Test Mode"=""} ("Result FGV Data In"), "Temp Chamber Name"=w301, "Test Description"=w300, "Project Name"=w299, "Test Phase"=w297, "Test Name"=w283, "Product Varient"=w284, "Product Name"=w280, "Schema"=w265, "Total No of Cycles"=w267, "Cycle Duration"=w278, "Current Cycle Number"=w268) -> (w305:T4)
                n142 = call "Result FGV.vi"("Action(Get All Data)"=Action_FGV."Set All Data", "error in"=w271, "Result FGV Data In"=w305) -> ("error out"=w290:errorcluster)  [unwired: 7 in, 1 out]
                n143 = property on="SchemaName" class="Str"(error in=w290, "Value"=w265) -> (error out=w289:errorcluster)  [unwired: 1 in, 1 out]
              }
            }
          }
          frame "Exit" {
            n144 = property class="SequenceContext"(reference=w338, error in=w333) -> (error out=w334:errorcluster, "Engine"=w339:refnum<k7>)  [unwired: 1 out]
            n145 = invoke class="IEngine" method="CommitGlobalsToDisk"(reference=w339, error in=w334, "promptOnSaveConflicts"=FALSE) -> (reference out=w335:refnum<k7>, error out=w336:errorcluster)  [unwired: 1 in, 2 out]
            n146 = Close Reference(reference=w335, error in (no error)=w336) -> (error out=w332:errorcluster)
          }
        }
        n147 = Compound Arithmetic op=OR(w28, w26) -> (w27:bool)
      }
    }
    frame Error {
    }
  }
  n148 = disable-structure shown="Enabled" {
    disable-tunnel: w8 -> [w345 w347]
    disable-tunnel: [w344 w347] -> w7
    frame Disabled {
      n149 = call "Database Driver.vi"("Options"=DB_Options."Close", "error in"=w345) -> ("error out"=w344:errorcluster)  [unwired: 6 in, 3 out]
    }
    frame Enabled {
    }
  }
  "error out" <- w7
